vi "Init DH20vi.vi"(8 "error in (no error)":errorcluster, 11 "Grove Thermocouple MCP9600 in":refnum<class "Grove Thermocouple MCP9600.lvclass">) -> (0 "error out":errorcluster, 3 "Grove Thermocouple MCP9600 out":refnum<class "Grove Thermocouple MCP9600.lvclass">)   [LabVIEW 2020, in "CTI-Peripheral.lvlib" / "Grove Thermocouple MCP9600.lvclass"]
uses:
  Grove Thermocouple MCP9600.lvclass
  Controls/ThermocoupleType.ctl
  Grove Thermocouple MCP9600.lvclass/Grove Thermocouple MCP9600.ctl
  CTI/I2C Connection/I2C Connection.lvclass/I2C Connection.ctl
  CTI/Session/I2C Write Data.vi
  CTI/Session/I2C Read Data.vi
  CTI/I2C Connection/I2C Connection.lvclass
panel:
  out "DeviceID":string
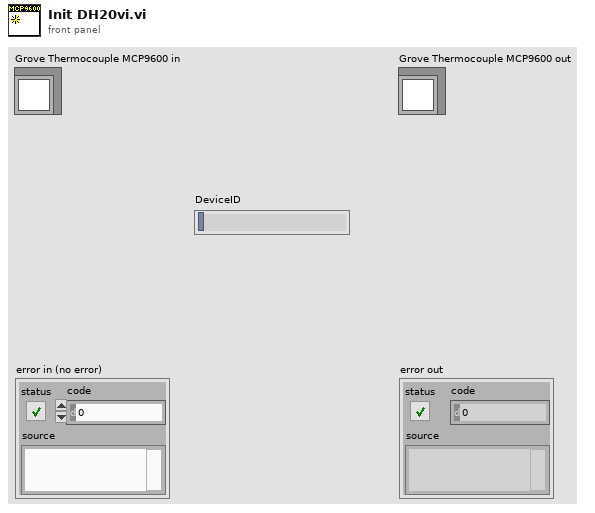
[diagram p1: front panel]
types:
  T1 = typedef "CTI-Peripheral.lvlib/Grove Thermocouple MCP9600.lvclass/ThermocoupleType.ctl" = enum16{"K", "J", "T", "N", "S", "E", "B", "R"}
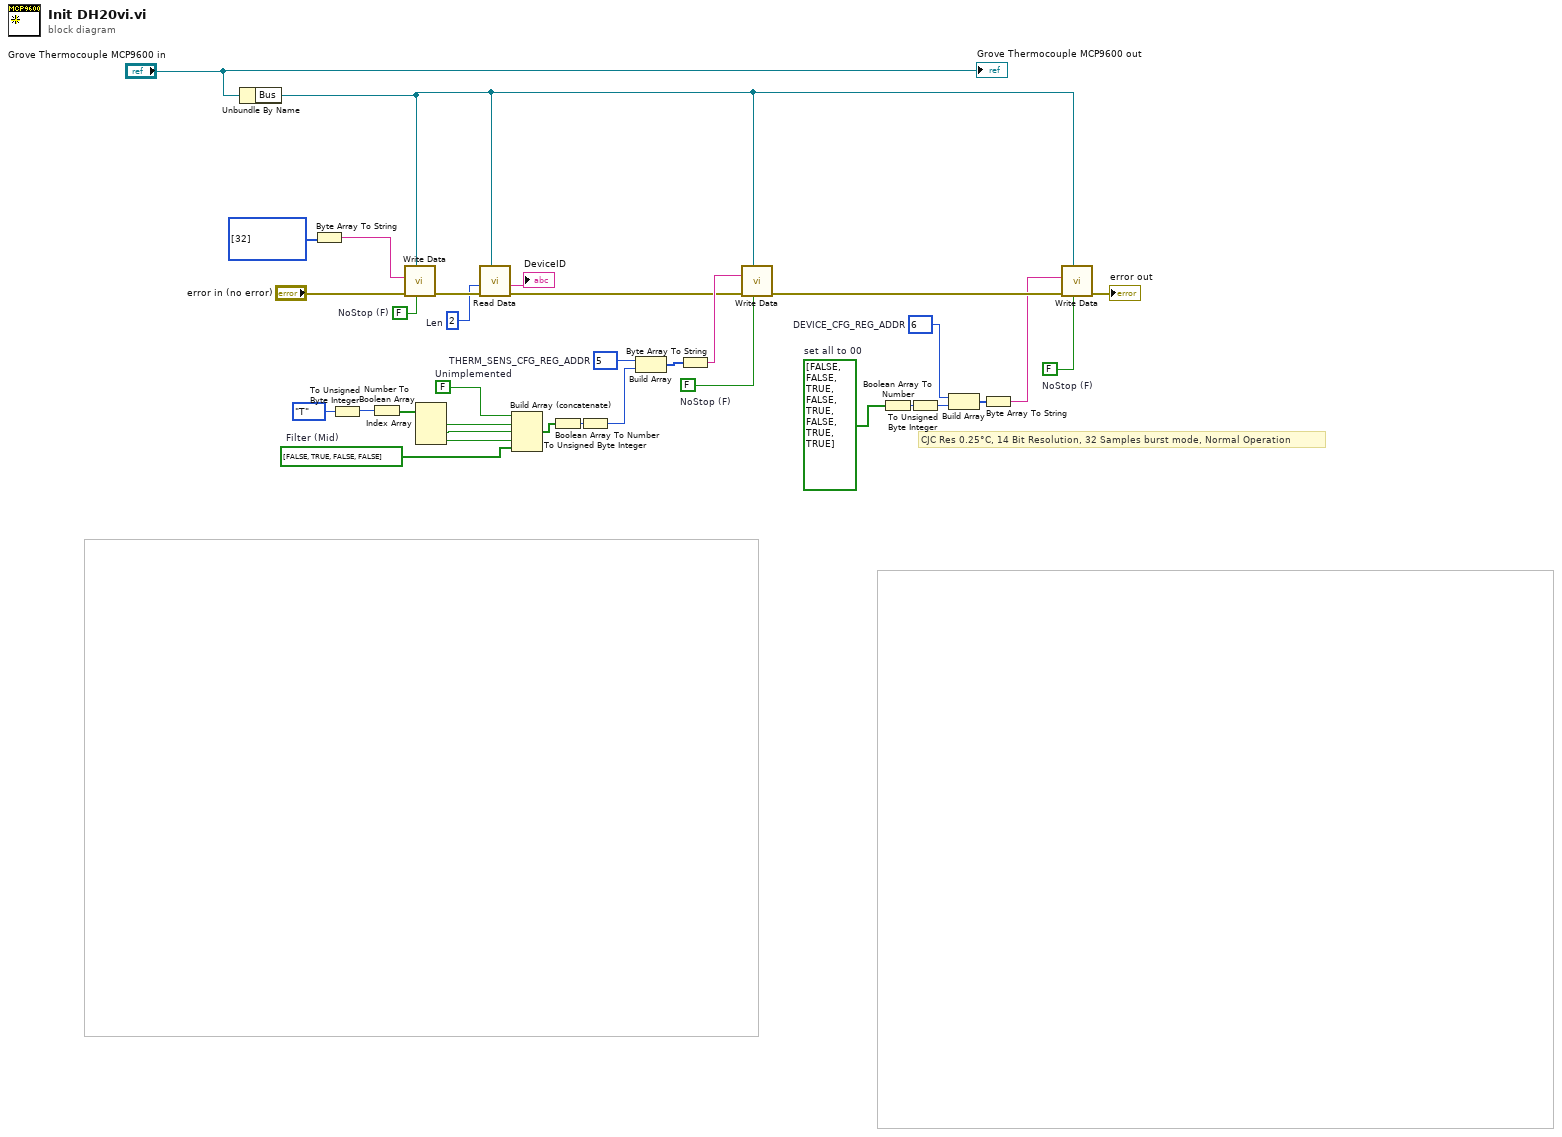
[diagram p0: block diagram]
diagram:
  w3 = FALSE  # NoStop (F)
  w8 = u8 2  # Len
  w15 = u8 6  # DEVICE_CFG_REG_ADDR
  w17 = bool[] [FALSE, FALSE, TRUE, FALSE, TRUE, FALSE, TRUE, TRUE]  # set all to 00
  w13 = bool[] [FALSE, TRUE, FALSE, FALSE]  # Filter (Mid)
  w22 = FALSE  # Unimplemented
  w29 = u8 5  # THERM_SENS_CFG_REG_ADDR
  w31 = FALSE  # NoStop (F)
  w33 = FALSE  # NoStop (F)
  # "CJC Res 0.25°C, 14 Bit Resolution, 32 Samples burst mode, Normal Operation"
  n1 = Unbundle By Name("Grove Thermocouple MCP9600 in") -> ("Bus"=w9:refnum<class "I2C Connection.lvclass">)
  n2 = Byte Array To String(unsigned byte array=u8[] [32] ("Start Register")) -> (string=w11:string)
  n3 = To Unsigned Byte Integer(number=ThermocoupleType."T" ("Thermocouple Type")) -> (unsigned 8bit integer=w27:u8)
  n4 = Number To Boolean Array(number=w27) -> (Boolean array=w26:bool[])
  n5 = call "Write Data.vi"("NoStop (F)"=w33, "I2C Connection"=w9, "error in (no error)"="error in (no error)", "Data"=w11) -> ("error out"=w10:errorcluster)  [unwired: 7 in]
  n6 = Index Array(array=w26) -> (element #1=w25:bool, element #2=w24:bool, element #3=w23:bool)  [unwired: 3 in]
  n7 = call "Read Data.vi"("I2C Connection"=w9, "error in (no error)"=w10, "Len"=w8) -> ("error out"=w5:errorcluster, "Data"=→"DeviceID":string)  [unwired: 7 in]
  n8 = Build Array (concatenate)(w22, w25, w24, w23, w13) -> (w21:bool[])
  n9 = Boolean Array To Number(Boolean array=w21) -> (number=w20:u32)
  n10 = To Unsigned Byte Integer(number=w20) -> (unsigned 8bit integer=w19:u8)
  n11 = Build Array(w29, w19) -> (w28:u8[])
  n12 = Byte Array To String(unsigned byte array=w28) -> (string=w6:string)
  n13 = call "Write Data.vi"("NoStop (F)"=w31, "I2C Connection"=w9, "error in (no error)"=w5, "Data"=w6) -> ("error out"=w4:errorcluster)  [unwired: 7 in]
  n14 = Boolean Array To Number(Boolean array=w17) -> (number=w18:u32)
  n15 = To Unsigned Byte Integer(number=w18) -> (unsigned 8bit integer=w16:u8)
  n16 = Build Array(w15, w16) -> (w14:u8[])
  n17 = Byte Array To String(unsigned byte array=w14) -> (string=w2:string)
  n18 = call "Write Data.vi"("NoStop (F)"=w3, "I2C Connection"=w9, "error in (no error)"=w4, "Data"=w2) -> ("error out"=→"error out":errorcluster)  [unwired: 7 in]
  "Grove Thermocouple MCP9600 out" <- "Grove Thermocouple MCP9600 in"
